vi "rvc Transformation Difference.vi"(10 "Final transformation":T1, 11 "Initial transformation":T1) -> (3 "Difference":dbl[](array[numeric]))   [LabVIEW 2013]
uses:
  <vilib>/Analysis/Matrix/Datatypes/RealMatrix.ctl
  <vilib>/Analysis/baseanly.llb/Real A x B.vi
  <vilib>/Analysis/7linalg.llb/Create Special Real Matrix.vi
  <vilib>/Analysis/Matrix/Numeric/Subtract/Subtract - RM,RM.vi
  <vilib>/robotics/Kinematics/NI_Kinematics.lvlib
  <vilib>/Analysis/NI_AALBase.lvlib
  <vilib>/Analysis/NI_AALPro.lvlib
  <vilib>/Analysis/Matrix/NI_Matrix.lvlib
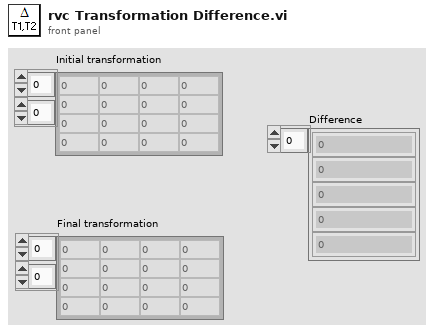
[diagram p1: front panel]
types:
  T1 = typedef "NI_Matrix.lvlib/RealMatrix.ctl" = dbl[][]
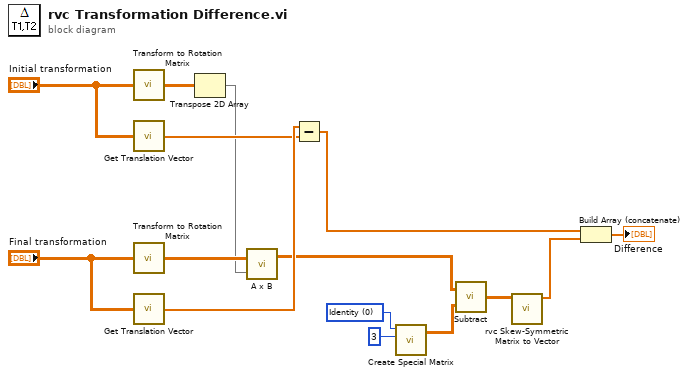
[diagram p0: block diagram]
diagram:
  w7 = 0 items=["Identity", "Diagonal", "Toeplitz", "Vandermonde", "Companion", "Hankel", "Hadamard", "Wilkinson", "Hilbert", "Inverse Hilbert", "Rosser", "Pascal"] ("matrix type")
  n1 = call <vilib>:"Transform to Rotation Matrix.vi"("transform"="Initial transformation") -> ("rotation matrix"=w11:T1)
  n2 = call <vilib>:"Get Translation Vector.vi"("transform"="Initial transformation") -> ("translation vector"=w12:dbl[])
  n3 = call <vilib>:"Transform to Rotation Matrix.vi"("transform"="Final transformation") -> ("rotation matrix"=w10:T1)
  n4 = call <vilib>:"Get Translation Vector.vi"("transform"="Final transformation") -> ("translation vector"=w13:dbl[])
  n5 = Transpose 2D Array(2D array=w11) -> (transposed array=w9:T1)
  n6 = call-poly <vilib>:"A x B.vi"("B"=w9, "A"=w10) -> ("A x B"=w5:T1)  [unwired: 1 out]
  n7 = Subtract(x=w13, y=w12) -> (x-y=w2:dbl[])
  n8 = call-poly <vilib>:"Create Special Matrix.vi"("matrix type"=w7, "matrix size"=3) -> ("Special Matrix"=w6:T1)  [unwired: 3 in, 1 out]
  n9 = call-poly <vilib>:"Subtract.vi"("Real Matrix B"=w6, "Real Matrix A"=w5) -> ("A - B"=w4:T1)
  n10 = call "rvc Skew-Symmetric Matrix to Vector.vi"("output variable in"=w4) -> ("output variable out"=w3:dbl[])  [unwired: 10 in]
  n11 = Build Array (concatenate)(w2, w3) -> (→"Difference":dbl[])
